vi "main_test.vi"() -> ()   [LabVIEW 2019]
uses:
  <vilib>/myRIO/Instrument Drivers/Onboard IO/I2C/typedefs/I2C Transfer Rate.ctl
  <vilib>/myRIO/Instrument Drivers/Onboard IO/I2C/I2C.lvlib
  <vilib>/myRIO/Instrument Drivers/Onboard IO/I2C/typedefs/I2C User Configuration.ctl
  <vilib>/myRIO/Instrument Drivers/Onboard IO/I2C/typedefs/I2C Configuration.ctl
  <vilib>/myRIO/Common/Instrument Driver Framework/myRIO v1.0/I2C/typedefs/I2C Channels Enum.ctl
  <vilib>/myRIO/Common/Instrument Driver Framework/Utilities/typedefs/Generic FPGA Reference.ctl
  <vilib>/myRIO/Common/Instrument Driver Framework/Utilities/typedefs/myRIO v1.0 Reference.ctl
  <vilib>/myRIO/Common/Instrument Driver Framework/Utilities/typedefs/Hardware Version Enum.ctl
  <vilib>/myRIO/Common/Instrument Driver Framework/Utilities/typedefs/myRIO Generic Hardware Reference.ctl
  <vilib>/myRIO/Instrument Drivers/Onboard IO/I2C/typedefs/I2C Reference.ctl
  <vilib>/myRIO/Instrument Drivers/Onboard IO/I2C/vis/Configure.vi
  <vilib>/userDefined/High Color/nirio_resource_hc.ctl
  <vilib>/myRIO/Common/Instrument Driver Framework/myRIO v1.0/I2C/vis/myRIO v1.1 Open I2C.vi
  <vilib>/myRIO/Instrument Drivers/Onboard IO/I2C/vis/myRIO I2C Open.xnode
  <vilib>/myRIO/Common/Instrument Driver Framework/Utilities/vis/Is FPGA Ref Available.vi
  <vilib>/myRIO/Express VI/Onboard IO/I2C/I2C Express VI.xnode
  <vilib>/Platform/TimedLoop/XDataNode/wakeup.ctl
  <vilib>/Platform/TimedLoop/XDataNode/XDNodeRunTimeDep.lvlib
  <vilib>/Platform/TimedLoop/XDataNode/nitl_modes.ctl
  <vilib>/Platform/TimedLoop/XDataNode/timing_clust.ctl
  <vilib>/platform/TimedLoop/XDataNode/XDataNode.xnode
  <vilib>/myRIO/Instrument Drivers/Onboard IO/I2C/vis/Write.vi
  <vilib>/myRIO/Instrument Drivers/Utilities/Utilities.lvlib
  <vilib>/myRIO/Instrument Drivers/Onboard IO/I2C/vis/Write Read.vi
  <vilib>/myRIO/Express VI/Onboard IO/PWM/PWM Express VI.xnode
  <vilib>/myRIO/Instrument Drivers/Onboard IO/PWM/vis/Set Duty Cycle and Frequency.vi
  <vilib>/myRIO/Instrument Drivers/Onboard IO/PWM/PWM.lvlib
  <vilib>/myRIO/Instrument Drivers/Onboard IO/PWM/typedefs/PWM Configuration.ctl
  <vilib>/myRIO/Common/Instrument Driver Framework/myRIO v1.0/PWM/typedefs/PWM Channels Enum.ctl
  <vilib>/myRIO/Instrument Drivers/Onboard IO/PWM/typedefs/PWM Reference.ctl
  <vilib>/myRIO/Instrument Drivers/Onboard IO/PWM/vis/myRIO PWM Open.xnode
  <vilib>/myRIO/Common/Instrument Driver Framework/myRIO v1.0/PWM/vis/myRIO v1.1 Open PWM.vi
  <vilib>/myRIO/Common/Instrument Driver Framework/myRIO v1.0/DIO/typedefs/DIO Channels Enum.ctl
  <vilib>/myRIO/Common/Instrument Driver Framework/myRIO v1.0/DIO/typedefs/DIO Channels List.ctl
  <vilib>/myRIO/Instrument Drivers/Onboard IO/DIO/typedefs/DIO Reference.ctl
  <vilib>/myRIO/Instrument Drivers/Onboard IO/DIO/DIO.lvlib
  <vilib>/myRIO/Instrument Drivers/Onboard IO/DIO/vis/Write.vi
  <vilib>/myRIO/Common/Instrument Driver Framework/myRIO v1.0/DIO/vis/myRIO v1.1 Open DIO.vi
  <vilib>/myRIO/Instrument Drivers/Onboard IO/DIO/vis/myRIO DIO Open.xnode
  <vilib>/myRIO/Express VI/Onboard IO/DO/DO Express VI.xnode
  <vilib>/imath/engines/lvmath2/RunTimeEngine/BuiltInFunctions/diag/NIMS_diag.vi
  <vilib>/imath/engines/lvmath2/RunTimeEngine/ErrorHandling/NIMS_Create Error From Enums.vi
  <vilib>/imath/engines/lvmath2/RunTimeEngine/NodeEndStatement/NIMS_NodeEndStatement_Output.vi
  <vilib>/imath/engines/lvmath2/RunTimeEngine/ErrorHandling/NIMS_Finalize Error.vi
  <instcachedir>/0/MCStatic_41946317732_460fc674ac509ba7029ac98c4ab25738_40677AF033AE4176B404E9AC0BBDDC84.lvgen/MCStatic_41946317732_460fc674ac509ba7029ac98c4ab25738_40677AF033AE4176B404E9AC0BBDDC84_001.vi
  <instcachedir>/0/MCStatic_41946317732_98df4686c37d1a1eae0c5985e9f7cbe2_A0FFC33B284B421AAD6E5346CB265B3A.lvgen/MCStatic_41946317732_98df4686c37d1a1eae0c5985e9f7cbe2_A0FFC33B284B421AAD6E5346CB265B3A_003.vi
  <instcachedir>/0/MCStatic_41946317732_460fc674ac509ba7029ac98c4ab25738_40677AF033AE4176B404E9AC0BBDDC84.lvgen/MCStatic_41946317732_460fc674ac509ba7029ac98c4ab25738_40677AF033AE4176B404E9AC0BBDDC84_003.vi
  <instcachedir>/0/MCStatic_41946317732_98df4686c37d1a1eae0c5985e9f7cbe2_A0FFC33B284B421AAD6E5346CB265B3A.lvgen/MCStatic_41946317732_98df4686c37d1a1eae0c5985e9f7cbe2_A0FFC33B284B421AAD6E5346CB265B3A_001.vi
  <vilib>/imath/engines/lvmath2/RunTimeEngine/BuiltInFunctions/length/NIMS_length(GV).vi
  <vilib>/imathl/engines/lvmath/Functions/Error Handling/Create Error.vi
  <vilib>/imath/engines/lvmath2/RunTimeEngine/BuiltInFunctions/ones/NIMS_V=ones(I32,I32).vi
  <vilib>/imath/engines/lvmath2/RunTimeEngine/RangeToken/NIMS_Range.vi
  OneDrive/Documents/LabVIEW Data/MathScriptVIs/MCStatic_41946317732_98df4686c37d1a1eae0c5985e9f7cbe2.vi
  <vilib>/imath/engines/lvmath2/RunTimeEngine/ArithmeticOperatorToken/NIMS_ArithmeticOperator_multmx.vi
  <vilib>/imath/engines/lvmath2/RunTimeEngine/BuiltInFunctions/max/1 input/NIMS_max(CM).vi
  <vilib>/imath/engines/lvmath/Functions/Error Handling/MergeErrorsWrapper.vi
  OneDrive/Documents/LabVIEW Data/MathScriptVIs/MCStatic_41946317732_460fc674ac509ba7029ac98c4ab25738.vi
  <vilib>/imath/engines/lvmath2/RunTimeEngine/ArithmeticOperatorToken/NIMS_ArithmeticOperator_minus.vi
  <vilib>/imath/engines/lvmath2/RunTimeEngine/BuiltInFunctions/norm/NIMS_norm(GM,DBL).vi
  <vilib>/imath/engines/lvmath2/RunTimeEngine/BuiltInFunctions/abs/NIMS_abs(signed).vi
  <vilib>/imath/engines/lvmath2/RunTimeEngine/BuiltInFunctions/max/1 input/NIMS_max(RM).vi
  <vilib>/imath/engines/lvmath2/RunTimeSupport/NIMS_Get Scalar_w Error.vi
  <vilib>/imath/engines/lvmath2/RunTimeEngine/BuiltInFunctions/eye/NIMS_M=eye(I32).vi
  <vilib>/imath/engines/lvmath2/RunTimeEngine/ArithmeticOperatorToken/NIMS_ArithmeticOperator_plus.vi
  <vilib>/imath/engines/lvmath2/RunTimeEngine/ArithmeticOperatorToken/NIMS_ArithmeticOperator_leftdivmx(C,C).vi
  <vilib>/imath/engines/lvmath2/RunTimeEngine/ArithmeticOperatorToken/NIMS_ArithmeticOperator_rightdiv.vi
  <vilib>/imath/engines/lvmath2/RunTimeEngine/ArithmeticOperatorToken/NIMS_ArithmeticOperator_rightdivmx(C,C).vi
  <vilib>/imath/engines/lvmath2/RunTimeEngine/ArithmeticOperatorToken/NIMS_ArithmeticOperator_powermx(M,M).vi
  <vilib>/imath/engines/lvmath2/RunTimeEngine/BuiltInFunctions/max/2 inputs/NIMS_max(CG,CG)-no size check.vi
  <vilib>/imath/engines/lvmath2/RunTimeEngine/CommandStatement/MC_CommandStatement_break.vi
  <vilib>/imath/engines/lvmath2/RunTimeEngine/CommandStatement/NIMS_CommandStatement_MaskErr.vi
  <vilib>/imath/engines/lvmath2/RunTimeEngine/NodeEndStatement/NIMS_NodeEndStatement_Get Vector.vi
  <vilib>/imath/engines/lvmath2/RunTimeEngine/BuiltInFunctions/mirrorh/NIMS_mirrorh(GM).vi
  <vilib>/imath/engines/lvmath2/RunTimeEngine/RowToken/NIMS_RowToken_M_M.vi
panel:
  in  "Count(mSec)":u32
  out "XY Graph":cluster{dbl[], dbl[]}[](graph)
  out "pm_hat_opt":dbl[](array[numeric])
  out "Late cycles":u16
  out "B_meas":dbl[](array[numeric])
  in  "Actuation on?":bool
  in  "Slide":dbl(slide) scale=-1.0..1.0
  in  "stop":bool
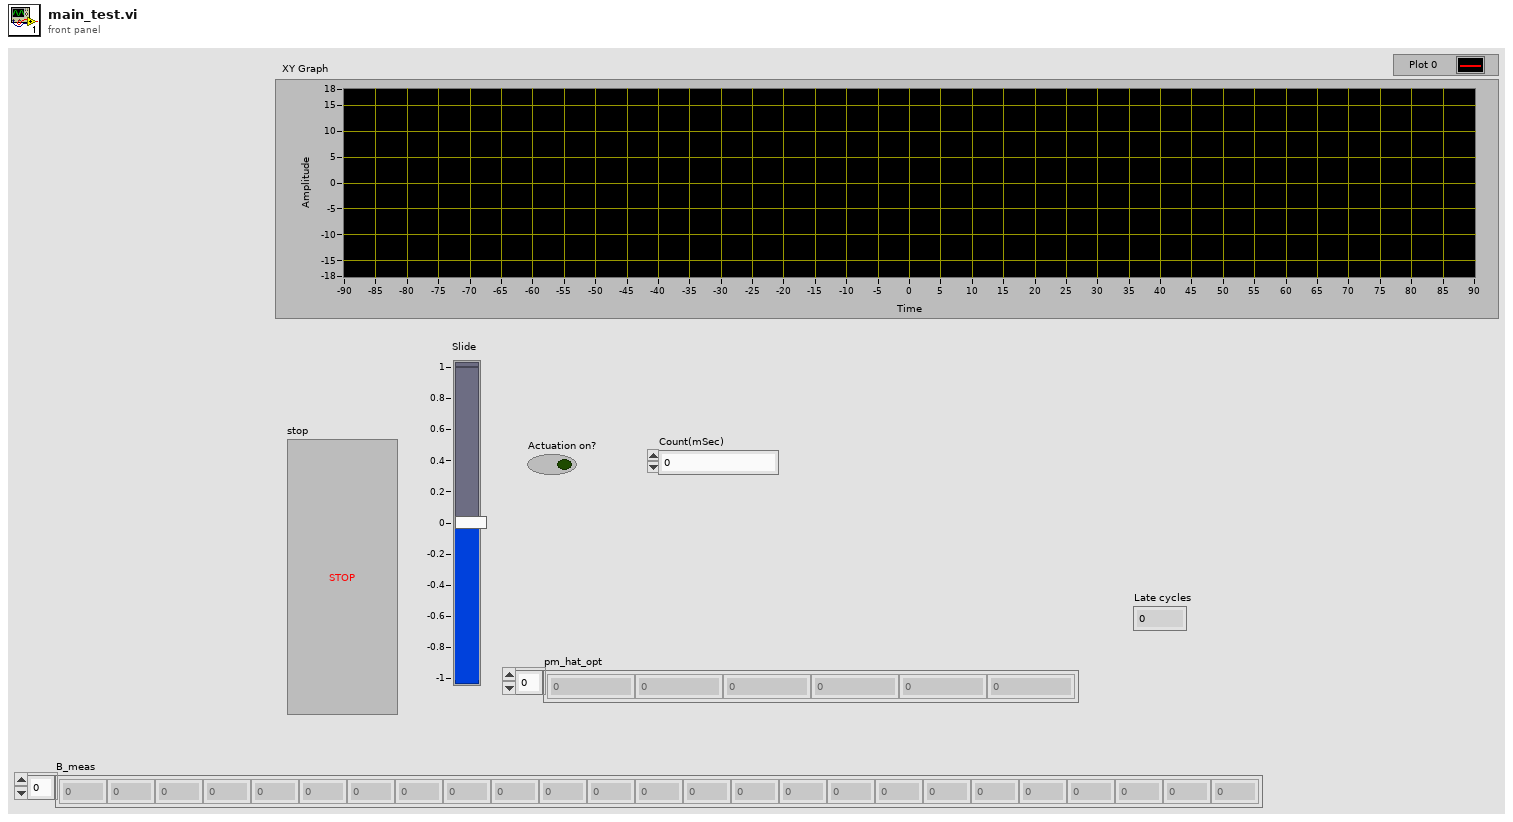
[diagram p1: front panel]
types:
  T1 = typedef "I2C.lvlib/I2C Reference.ctl" = cluster{"myRIO Reference":T2, "I2C Channels Enum":T6, "I2C Configuration":T7}
  T2 = typedef "myRIO Generic Hardware Reference.ctl" = cluster{"myRIO Model":T3, "myRIO Hardware Reference":T4}
  T3 = typedef "Hardware Version Enum.ctl" = enum16{"Unknown", "myRIO-1900", "myRIO-1950", "roboRIO", "NI ELVIS RIO CM", "ELVIS III"}
  T4 = typedef "myRIO v1.0 Reference.ctl" = cluster{"Generic FPGA Reference":T5, "Allow multiple opens":bool}
  T5 = typedef "Generic FPGA Reference.ctl" = refnum<k20>
  T6 = typedef "I2C Channels Enum.ctl" = enum16{"Not Connected", "A/I2C", "B/I2C", "I2C/I2C"}
  T7 = typedef "I2C.lvlib/I2C Configuration.ctl" = cluster{"I2C Transfer Rate":T8}
  T8 = typedef "I2C.lvlib/I2C Transfer Rate.ctl" = enum16{"Standard mode (100 kbps)", "Fast mode (400 kbps)"}
  T9 = typedef "I2C.lvlib/I2C User Configuration.ctl" = cluster{"I2C Transfer Rate":T8}
  T10 = typedef "nirio_resource_hc.ctl" = tag
  T11 = typedef "DIO.lvlib/DIO Reference.ctl" = cluster{"myRIO Reference":T2, "DIO Channels List":T12}
  T12 = typedef "DIO Channels List.ctl" = T13[]
  T13 = typedef "DIO Channels Enum.ctl" = enum16{"Not Connected", "C/DIO0", "C/DIO1", "C/DIO2", "C/DIO3", "C/DIO4", "C/DIO5", "C/DIO6", "C/DIO7", "A/DIO0", "A/DIO1", "A/DIO2", "A/DIO3", "A/DIO4", "A/DIO5", "A/DIO6", "A/DIO7", "A/DIO8", "A/DIO9", "A/DIO10", "A/DIO11", "A/DIO12", "A/DIO13", "A/DIO14", "A/DIO15", "A/DIO16", "A/DIO17", "A/DIO18", "A/DIO19", "B/DIO0", "B/DIO1", "B/DIO2", "B/DIO3", "B/DIO4", "B/DIO5", "B/DIO6", "B/DIO7", "B/DIO8", "B/DIO9", "B/DIO10", "B/DIO11", "B/DIO12", "B/DIO13", "B/DIO14", "B/DIO15", "B/DIO16", "B/DIO17", "B/DIO18", "B/DIO19", "LED0", "LED1", "LED2", "LED3", "Button0", "DIO/DIO0", "DIO/DIO1", "DIO/DIO2", "DIO/DIO3", "DIO/DIO4", "DIO/DIO5", "DIO/DIO6", "DIO/DIO7", "DIO/DIO8", "DIO/DIO9", "SPI/CS0", "SPI/CS1", "SPI/CS2", "SPI/CS3", "LED RADIO (Green)", "LED RADIO (Red)", "LED COMM (Green)", "LED COMM (Red)", "LED MODE (Green)", "LED MODE (Red)"}
  T14 = typedef "PWM.lvlib/PWM Reference.ctl" = cluster{"myRIO Reference":T2, "PWM Channels Enum":T15, "PWM Configuration":T16}
  T15 = typedef "PWM Channels Enum.ctl" = enum16{"Not Connected", "C/PWM0", "C/PWM1", "A/PWM0", "A/PWM1", "A/PWM2", "A/PWM3", "A/PWM4", "A/PWM5", "A/PWM6", "A/PWM7", "A/PWM8", "A/PWM9", "A/PWM10", "A/PWM11", "A/PWM12", "A/PWM13", "A/PWM14", "A/PWM15", "A/PWM16", "A/PWM17", "A/PWM18", "A/PWM19", "B/PWM0", "B/PWM1", "B/PWM2", "B/PWM3", "B/PWM4", "B/PWM5", "B/PWM6", "B/PWM7", "B/PWM8", "B/PWM9", "B/PWM10", "B/PWM11", "B/PWM12", "B/PWM13", "B/PWM14", "B/PWM15", "B/PWM16", "B/PWM17", "B/PWM18", "B/PWM19", "PWM/PWM0", "PWM/PWM1", "PWM/PWM2", "PWM/PWM3", "PWM/PWM4", "PWM/PWM5", "PWM/PWM6", "PWM/PWM7", "PWM/PWM8", "PWM/PWM9"}
  T16 = typedef "PWM.lvlib/PWM Configuration.ctl" = cluster{"Frequency":dbl, "Duty Cycle":dbl}
  T17 = typedef "XDNodeRunTimeDep.lvlib/timing_clust.ctl" = cluster{"Expected End [f-1]":u64, "Actual End [f-1]":u64, "Finished Late? [f-1]":bool, "Expected End [i-1]":u64, "Actual End [i-1]":u64, "Finished Late? [i-1]":bool, "Expected Start [i]":u64, "Actual Start [i]":u64, "Expected Start [f]":u64, "Actual Start [f]":u64, "Source Name":string, "Structure Name":string, "Period":i64, "Deadline":i64, "Offset":i64, "Start":i64, "Priority":i32, "Timeout":i32, "Mode":T18, "Wakeup Reason":T19, "Error":errorcluster, "Source Type":string, "Secondary Source Type":string, "Global End Time":u64, "Global Start Time":u64, "Frame Duration":u64, "Iteration Duration":u64, "Assigned CPU":i32, "I/O Scan Engine Mode":u32}
  T18 = typedef "XDNodeRunTimeDep.lvlib/nitl_modes.ctl" = enum32{"No Change", "Process missed periods, maintain original phase", "Discard missed periods, maintain original phase", "Process missed periods, ignore original phase", "Discard missed periods, ignore original phase"}
  T19 = typedef "XDNodeRunTimeDep.lvlib/wakeup.ctl" = enum32{"Normal", "Aborted", "Asynchronous wakeup", "Timing source error", "Timed loop error", "Timeout"}
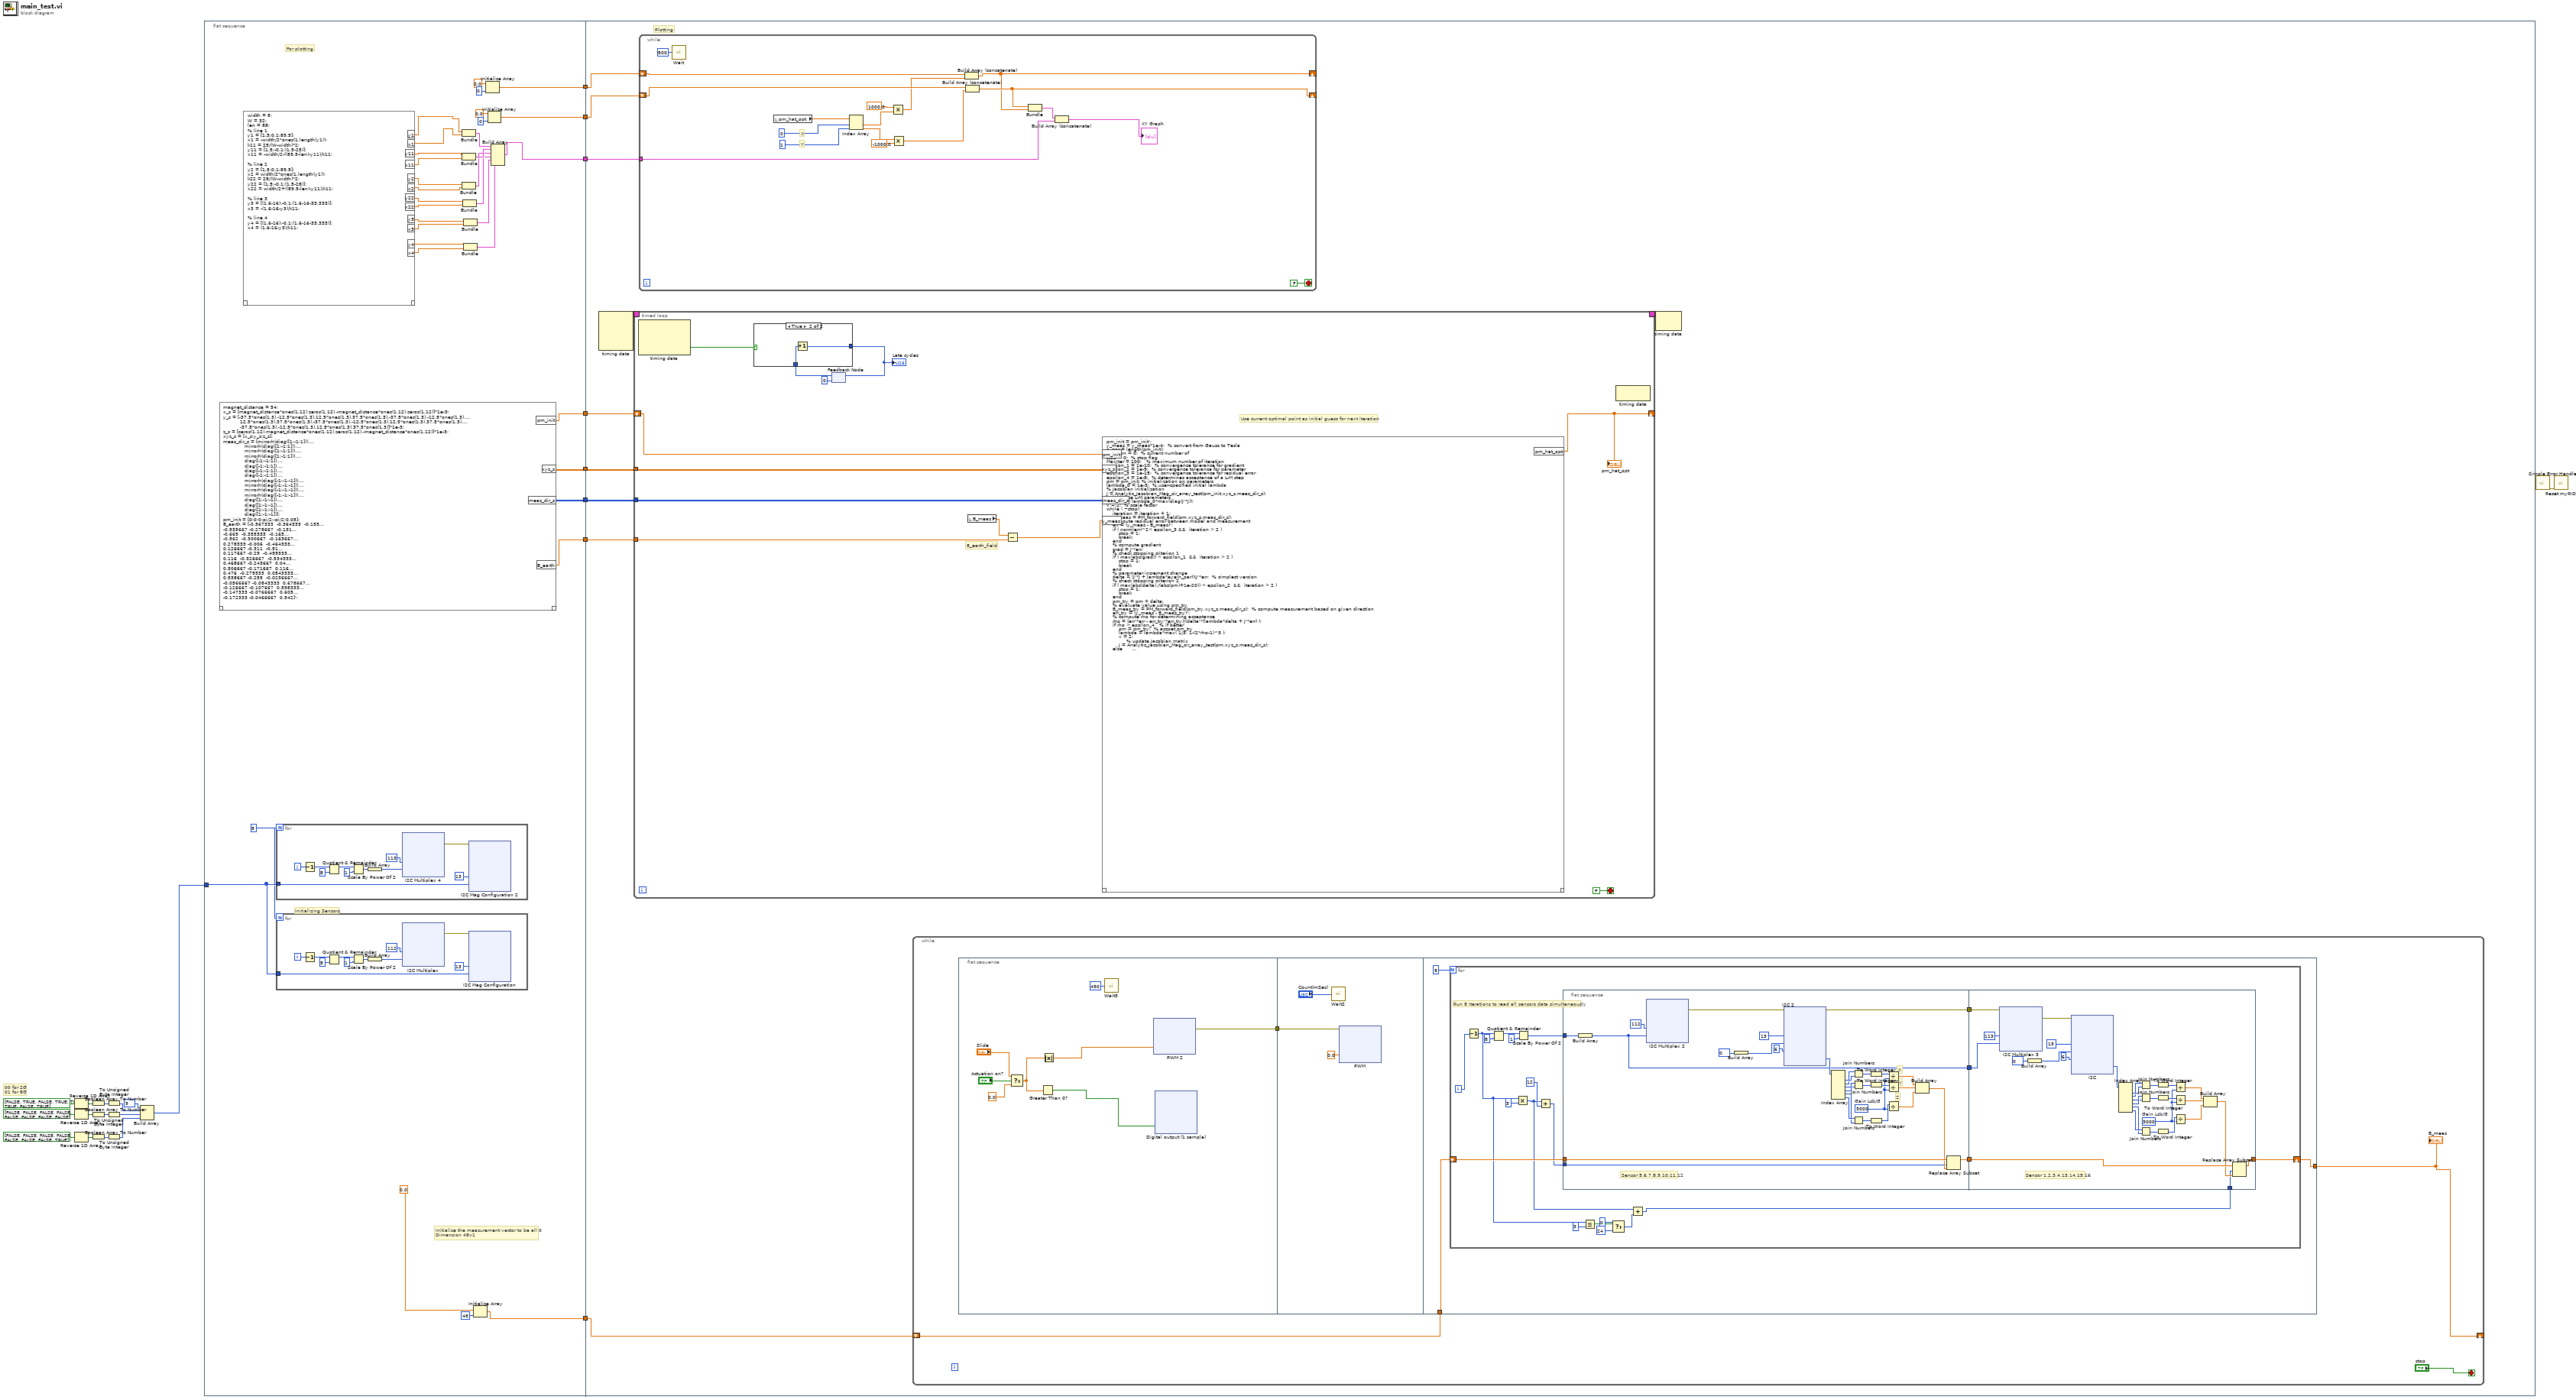
[diagram p0: block diagram]
diagram:
  # "00 for 2G\n01 for 8G"
  n1 = Reverse 1D Array(array=bool[] [FALSE, TRUE, FALSE, TRUE, TRUE, TRUE, FALSE, TRUE]) -> (reversed array=w22:bool[])
  n2 = Reverse 1D Array(array=bool[] [FALSE, FALSE, FALSE, FALSE, FALSE, FALSE, FALSE, FALSE]) -> (reversed array=w21:bool[])
  n3 = Reverse 1D Array(array=bool[] [FALSE, FALSE, FALSE, FALSE, FALSE, FALSE, FALSE, TRUE]) -> (reversed array=w19:bool[])
  n4 = Boolean Array To Number(Boolean array=w22) -> (number=w16:u32)
  n5 = Boolean Array To Number(Boolean array=w21) -> (number=w15:u32)
  n6 = Boolean Array To Number(Boolean array=w19) -> (number=w14:u32)
  n7 = To Unsigned Byte Integer(number=w16) -> (unsigned 8bit integer=w13:u8)
  n8 = To Unsigned Byte Integer(number=w15) -> (unsigned 8bit integer=w12:u8)
  n9 = To Unsigned Byte Integer(number=w14) -> (unsigned 8bit integer=w11:u8)
  n10 = Build Array(u8 9 ("address"), w13, w12, w11) -> (w10:u8[])
  n11 = flat-sequence {
    tunnel: w10 -> [w57]
    tunnel: [w55] -> w8
    tunnel: [w54] -> w7
    tunnel: [w51] -> w6
    tunnel: [w50] -> w5
    tunnel: [w49] -> w4
    tunnel: [w44] -> w3
    tunnel: [w43] -> w2
    tunnel: [w24] -> w1
    tunnel: w8 -> [w784]
    tunnel: w7 -> [w783]
    tunnel: w6 -> [w780]
    tunnel: w5 -> [w779]
    tunnel: w4 -> [w778]
    tunnel: w3 -> [w777]
    tunnel: w2 -> [w776]
    tunnel: w1 -> [w775]
    frame #0 {
      w56 = 8
      # "For plotting"
      # "Initialize the measurement vector to be all 0\nDimension 48x1"
      # "Initializing Sensors"
      n12 = mathscript code="magnet_distance = 54;\nx_s = [magnet_distance*ones(1,12),zeros(1,12),-magnet_distance*ones(1,12),zeros(1,12)]*1e-3; \ny_s = [-37.5*ones(1,3),-12.5*ones(1,3),12.5*ones(1,3),37.5*ones(1,3),-37.5*ones(1,3),-12.5*ones(1,3),...\n           12.5*ones(1,3),37.5*ones(1,3),-37.5*ones(1,3),-12.5*ones(1,3),12.5*ones(1,3),37.5*ones(1,3),...\n           -37.5*ones(1,3),-12.5*ones(1,3),12.5*ones(1,3),37.5*ones(1,3)]*1e-3; \nz_s = [zeros(1,12),magnet_distance*ones(1,12),zeros(1,12),-magnet_distance*ones(1,12)]*1e-3; \nxyz_s = [x_s;y_s;z_s];  \nmeas_dir_s = [mirrorh(diag([1;-1;1])),...\n              mirrorh(diag([1;-1;1])),...\n              mirrorh(diag([1;-1;1])),...\n              mirrorh(diag([1;-1;1])),...\n              diag([-1;-1;1]),...\n              diag([-1;-1;1]),...\n              diag([-1;-1;1]),...\n              diag([-1;-1;1]),...\n              mirrorh(diag([-1;-1;-1])),...\n              mirrorh(diag([-1;-1;-1])),...\n              mirrorh(diag([-1;-1;-1])),...\n              mirrorh(diag([-1;-1;-1])),... \n              diag([1;-1;-1]),...\n              diag([1;-1;-1]),...\n              diag([1;-1;-1]),...\n              diag([1;-1;-1])];\npm_init = [0;0;0;pi/2;-pi/2;0.05];\nB_earth = [-0.567333\t\t-0.364333\t\t-0.155...\n-0.535667\t-0.278667\t\t-0.131...\n-0.669\t\t-0.355333\t\t-0.165...\n-0.562\t\t-0.300667\t\t-0.163667...\n0.278333\t-0.006\t\t-0.464333...\n0.126667\t-0.311\t\t-0.51...\n0.117667\t-0.29\t\t-0.499333...\n0.116\t\t-0.326667\t\t-0.534333...\n0.468667\t-0.243667\t\t0.04...\n0.506667\t-0.171667\t\t0.116...\n0.476\t\t-0.279333\t\t0.0543333...\n0.538667\t-0.255\t\t-0.0236667...\n-0.0566667\t-0.0843333\t\t0.678667...\n-0.126667\t-0.107667\t\t0.598333...\n-0.147333\t-0.0766667\t\t0.605...\n-0.172333\t-0.0466667\t\t0.542]';"() -> ("meas_dir_s"=w55:i32[][], "xyz_s"=w54:dbl[][], "pm_init"=w50:dbl[], "B_earth"=w49:dbl[])  [unwired: 1 in, 1 out]
      n13 = mathscript code="width = 8;\nW = 32;\nlen = 88;\n% line 1\ny1 = [1.5:0.1:89.5];\nx1 = -width/2*ones(1,length(y1));\nk11 = 25/(W-width)*2;\ny11 = [1.5:-0.1:(1.5-25)];\nx11 = -width/2-((89.5-len)-y11)/k11;\n\n% line 2\ny2 = [1.5:0.1:89.5];\nx2 = width/2*ones(1,length(y1));\nk22 = 28/(W-width)*2;\ny22 = [1.5:-0.1:(1.5-28)];\nx22 = width/2+((89.5-len)-y11)/k11;\n\n% line 3\ny3 = [(1.6-16):-0.1:(1.6-16-33.333)];\nx3 = -(1.6-16-y3)/k11;\n\n% line 4\ny4 = [(1.6-16):-0.1:(1.6-16-33.333)];\nx4 = (1.6-16-y3)/k11;"() -> ("y1"=w42:dbl[], "x1"=w41:dbl[], "y11"=w40:dbl[], "x11"=w39:dbl[], "y2"=w36:dbl[], "x2"=w35:dbl[], "y22"=w33:dbl[], "x22"=w32:dbl[], "y3"=w30:dbl[], "x3"=w29:dbl[], "y4"=w27:dbl[], "x4"=w26:dbl[])  [unwired: 1 in, 1 out]
      n14 = for {
        N: w56 -> [_]
        tunnel: w57 -> [w608]
        i -> [w602]
        n15 = Decrement(x=w602) -> (x-1=w601:i32)
        n16 = Quotient & Remainder(x=w601, y=8) -> (x-y*floor(x/y)=w603:i32)  [unwired: 1 out]
        n17 = Scale By Power Of 2(n=w603, x=1) -> (x*2^n=w605:i32)
        n18 = Build Array(w605) -> (w611:i32[])
        n19 = xnode "I2C Multiplex 4"("Slave Address (7-bit)"=u8 113, "Bytes to Write"=w611) -> ("error out"=w610:errorcluster)  [unwired: 1 in]
        n20 = xnode "I2C Mag Configuration 2"("Slave Address (7-bit)"=u8 13, "Bytes to Write"=w608, "error in (no error)"=w610) -> ()  [unwired: 1 out]
      }
      n21 = for {
        N: w56 -> [_]
        tunnel: w57 -> [w695]
        i -> [w689]
        n22 = Decrement(x=w689) -> (x-1=w688:i32)
        n23 = Quotient & Remainder(x=w688, y=8) -> (x-y*floor(x/y)=w690:i32)  [unwired: 1 out]
        n24 = Scale By Power Of 2(n=w690, x=1) -> (x*2^n=w692:i32)
        n25 = Build Array(w692) -> (w698:i32[])
        n26 = xnode "I2C Multiplex"("Slave Address (7-bit)"=u8 112, "Bytes to Write"=w698) -> ("error out"=w697:errorcluster)  [unwired: 1 in]
        n27 = xnode "I2C Mag Configuration"("Slave Address (7-bit)"=u8 13, "Bytes to Write"=w695, "error in (no error)"=w697) -> ()  [unwired: 1 out]
      }
      n28 = Bundle("y2"=w36, "x2"=w35) -> (w34:cluster{"y2":dbl[], "x2":dbl[]})  [unwired: 1 in]
      n29 = Bundle("y1"=w42, "x1"=w41) -> (w38:cluster{"y1":dbl[], "x1":dbl[]})  [unwired: 1 in]
      n30 = Bundle("y11"=w40, "x11"=w39) -> (w37:cluster{"y11":dbl[], "x11":dbl[]})  [unwired: 1 in]
      n31 = Bundle("y22"=w33, "x22"=w32) -> (w31:cluster{"y22":dbl[], "x22":dbl[]})  [unwired: 1 in]
      n32 = Bundle("y3"=w30, "x3"=w29) -> (w28:cluster{"y3":dbl[], "x3":dbl[]})  [unwired: 1 in]
      n33 = Bundle("y4"=w27, "x4"=w26) -> (w25:cluster{"y4":dbl[], "x4":dbl[]})  [unwired: 1 in]
      n34 = Initialize Array(0.0 ("element"), 48 ("dimension size")) -> (w51:dbl[])
      n35 = Initialize Array(0.0 ("element"), 0 ("dimension size")) -> (w44:dbl[])
      n36 = Initialize Array(0.0 ("element"), 0 ("dimension size")) -> (w43:dbl[])
      n37 = Build Array(w38, w37, w34, w31, w28, w25) -> (w24:cluster{"y4":dbl[], "x4":dbl[]}[])
    }
    frame #1 {
      # "Plotting"
      n38 = node-c288() -> (w782:T17)  [unwired: 4 in]
      n39 = timed-loop {
        tunnel: w784 -> [w1173]
        tunnel: w783 -> [w1172]
        timing: w782 -> [_]
        timing-out: [_] -> w781
        shift-right: [w1165] -> _
        shift-left: w779 -> [w1166]
        tunnel: w778 -> [w1163]
        stop <- FALSE stop-if-true
        # "B_earth_field"
        # "Use current optimal point as initial guess for next iteration"
        n40 = node-c288() -> (w1167:bool)  [unwired: 1 in, 3 out]
        n41 = feedback #1(u16 0) -> (w1170:u16)
        n42 = case shown="True" w1167 {
          tunnel: w1170 -> [w1174 w1176]
          tunnel: [w1174 w1175] -> w1169
          frame False {
          }
          frame True {
            n43 = Increment(x=w1176) -> (x+1=w1175:u16)
          }
        }
        "Late cycles" <- w1169
        n44 = feedback-in #1(w1169) -> ()
        n45 = local read "B_meas"() -> (w1164:dbl[])
        n46 = Subtract(x=w1164, y=w1163) -> (x-y=w1162:dbl[])
        n47 = mathscript code="pm_init = pm_init';\ny_meas = y_meas*1e-4;  % convert from Gauss to Tesla\nn_par = length(pm_init);\niteration = 0;  % current number of \nstop = 0;  % stop flag\nMaxIter = 100;   % maximum number of iteration\nepsilon_1 = 1e-10;  % convergence tolerance for gradient\nepsilon_2 = 1e-9;  % convergence tolerance for parameter\nepsilon_3 = 1e-15;  % convergence tolerance for residual error\nepsilon_4 = 1e-8;  % determines acceptance of a L-M step\npm = pm_init; % initialization on parameters\nlambda_0 = 1e-3;  % user-specified initial lambda\n% Jacobian initialization\nJ = Analytic_Jacobian_Mag_cir_array_test(pm_init,xyz_s,meas_dir_s);\n% initialize L-M parameters\nlambda = lambda_0*max(diag(J'*J));\nv = 2;  % scale factor\nwhile ( ~stop)\n    iteration = iteration + 1;\n    B_meas = PM_forward_field(pm,xyz_s,meas_dir_s);\n% compute residual error between model and measurement\n    err = (y_meas - B_meas)';\n    if ( norm(err)^2< epsilon_3 &&  iteration > 2 )\n        stop = 1;\n        break;\n    end\n    % compute gradient\n    grad = J'*err;\n    % check stopping criterion 1\n    if ( max(abs(grad)) < epsilon_1  &&  iteration > 2 )\n        stop = 1;\n        break\n    end\n    % parameter increment change\n    delta = (J'*J + lambda*eye(n_par))\\J'*err;  % simplest version\n    % check stopping criterion 2 \n    if ( max(abs(delta)./(abs(pm)+1e-20)) < epsilon_2  &&  iteration > 2 )\n        stop = 1;\n        break\n    end\n    pm_try = pm + delta;\n    % evaluate value using pm_try\n    B_meas_try = PM_forward_field(pm_try,xyz_s,meas_dir_s);  % compute measurement based on given direction\n    err_try = (y_meas - B_meas_try)';\n    % compute rho for determining acceptance\n    rho = (err'*err - err_try'*err_try)/(delta'*(lambda*delta + J'*err) );\n    if rho > epsilon_4   % if better\n        pm = pm_try;  % accpet pm_try\n        lambda = lambda*max( 1/3, 1-(2*rho-1)^3 );\n        v = 2;\n             % update Jacobian matrix\n        J = Analytic_Jacobian_Mag_cir_array_test(pm,xyz_s,meas_dir_s);\n    else      % if not better\n        lambda = lambda*v;\n        v = 2*v;\n    end\n    if ( iteration == MaxIter )\n        stop = 1;\n    end\nend\n\npm_hat_opt = pm;"("meas_dir_s"=w1173, "xyz_s"=w1172, "y_meas"=w1162, "pm_init"=w1166) -> ("pm_hat_opt"=w1165:dbl[])  [unwired: 1 in, 1 out]
        "pm_hat_opt" <- w1165
        n48 = node-c288() -> ()  [unwired: 1 in, 1 out]
      }
      n49 = while {
        shift-right: [w1153] -> _
        shift-left: w777 -> [w1156]
        shift-right: [w1154] -> _
        shift-left: w776 -> [w1155]
        tunnel: w775 -> [w1144]
        stop <- FALSE stop-if-true
        # "X"
        # "Y"
        n50 = call "Wait"("Count(mSec)"=u32 500) -> ()  [unwired: 1 out]
        n51 = local read "pm_hat_opt"() -> (w1160:dbl[])
        n52 = Index Array(array=w1160, index #1=0 ("index"), index #2=1 ("index")) -> (element #1=w1149:dbl, element #2=w1152:dbl)
        n53 = Multiply(x=1000.0, y=w1149) -> (x*y=w1147:dbl)
        n54 = Multiply(x=w1152, y=-1000.0) -> (x*y=w1150:dbl)
        n55 = Build Array (concatenate)(w1156, w1147) -> (w1153:dbl[])
        n56 = Build Array (concatenate)(w1155, w1150) -> (w1154:dbl[])
        n57 = Bundle(w1154, w1153) -> (w1145:cluster{dbl[], dbl[]})  [unwired: 1 in]
        n58 = Build Array (concatenate)(w1145, w1144) -> (→"XY Graph":cluster{"y4":dbl[], "x4":dbl[]}[])
      }
      n59 = while {
        shift-right: [w785] -> _
        shift-left: w780 -> [w786]
        stop <- "stop" stop-if-true
        n60 = flat-sequence {
          tunnel: [w795] -> w787
          tunnel: w787 -> [w868]
          tunnel: w786 -> [w906]
          tunnel: [w905] -> w785
          frame #0 {
            n61 = Select(t="Slide", s="Actuation on?", f=0.0) -> (s? t:f=w790:dbl)
            n62 = Greater Than 0?(x=w790) -> (x > 0?=w789:bool)
            n63 = Absolute Value(x=w790) -> (abs(x)=w791:dbl)
            n64 = call "Wait3"("Count(mSec)"=u32 490) -> ()  [unwired: 1 out]
            n65 = xnode "PWM 2"("Duty Cycle"=w791) -> ("error out"=w795:errorcluster)  [unwired: 1 in]
            n66 = xnode "Digital output (1 sample)"("C/DIO2 (DIO2)"=w789) -> ()  [unwired: 1 in, 1 out]
          }
          frame #1 {
            n67 = call "Wait2"("Count(mSec)"="Count(mSec)") -> ()  [unwired: 1 out]
            n68 = xnode "PWM"("Duty Cycle"=0.0, "error in (no error)"=w868) -> ()  [unwired: 1 out]
          }
          frame #2 {
            # "Run 8 Iterations to read all sensors data simultaneously"
            n69 = for {
              N: 8 -> [_]
              shift-right: [w919] -> w905
              shift-left: w906 -> [w921]
              i -> [w922]
              n70 = Decrement(x=w922) -> (x-1=w915:i32)
              n71 = Quotient & Remainder(x=w915, y=8) -> (x-y*floor(x/y)=w923:i32)  [unwired: 1 out]
              n72 = Multiply(x=w915, y=3) -> (x*y=w912:i32)
              n73 = Scale By Power Of 2(n=w923, x=1) -> (x*2^n=w924:i32)
              n74 = Add(x=w912, y=12) -> (x+y=w916:i32)
              n75 = flat-sequence {
                tunnel: w926 -> [w939]
                tunnel: [w939] -> w929
                tunnel: [w937] -> w928
                tunnel: w921 -> [w933]
                tunnel: [w932] -> w920
                tunnel: w916 -> [w930]
                tunnel: w929 -> [w1046]
                tunnel: w928 -> [w1044]
                tunnel: w920 -> [w1043]
                tunnel: [w1042] -> w919
                tunnel: w908 -> [w1037]
                frame #0 {
                  w948 = i16 3000  # Gain Lsb/G
                  # "Sensor 5,6,7,8,9,10,11,12"
                  # "Z"
                  # "Y"
                  # "X"
                  n76 = xnode "I2C Multiplex 2"("Slave Address (7-bit)"=u8 112, "Bytes to Write"=w939) -> ("error out"=w938:errorcluster)  [unwired: 1 in]
                  n77 = Build Array(u8 0) -> (w952:u8[])
                  n78 = xnode "I2C 2"("Slave Address (7-bit)"=u8 13, "Bytes to Write"=w952, "Byte Count"=u32 6, "error in (no error)"=w938) -> ("Bytes Read"=w955:u8[], "error out"=w937:errorcluster)
                  n79 = Index Array(array=w955) -> (element #1=w947:u8, element #2=w946:u8, element #3=w944:u8, element #4=w945:u8, element #5=w942:u8, element #6=w943:u8)  [unwired: 6 in]
                  n80 = Join Numbers(hi=w946, lo=w947) -> ((hi.lo)=w958:u16)
                  n81 = Join Numbers(hi=w945, lo=w944) -> ((hi.lo)=w956:u16)
                  n82 = Join Numbers(hi=w943, lo=w942) -> ((hi.lo)=w957:u16)
                  n83 = To Word Integer(number=w958) -> (16bit integer=w951:i16)
                  n84 = To Word Integer(number=w956) -> (16bit integer=w950:i16)
                  n85 = To Word Integer(number=w957) -> (16bit integer=w949:i16)
                  n86 = Divide(x=w951, y=w948) -> (x/y=w936:dbl)
                  n87 = Divide(x=w950, y=w948) -> (x/y=w935:dbl)
                  n88 = Divide(x=w949, y=w948) -> (x/y=w934:dbl)
                  n89 = Build Array(w936, w935, w934) -> (w931:dbl[])
                  n90 = Replace Array Subset(array=w933, new element=w931, index=w930) -> (w932:dbl[])
                }
                frame #1 {
                  w1055 = i16 3000  # Gain Lsb/G
                  # "Sensor 1,2,3,4,13,14,15,16"
                  n91 = xnode "I2C Multiplex 3"("Slave Address (7-bit)"=u8 113, "Bytes to Write"=w1046, "error in (no error)"=w1044) -> ("error out"=w1045:errorcluster)
                  n92 = Build Array(u8 0) -> (w1059:u8[])
                  n93 = xnode "I2C"("Slave Address (7-bit)"=u8 13, "Bytes to Write"=w1059, "Byte Count"=u32 6, "error in (no error)"=w1045) -> ("Bytes Read"=w1062:u8[])  [unwired: 1 out]
                  n94 = Index Array(array=w1062) -> (element #1=w1054:u8, element #2=w1053:u8, element #3=w1051:u8, element #4=w1052:u8, element #5=w1049:u8, element #6=w1050:u8)  [unwired: 6 in]
                  n95 = Join Numbers(hi=w1053, lo=w1054) -> ((hi.lo)=w1065:u16)
                  n96 = Join Numbers(hi=w1052, lo=w1051) -> ((hi.lo)=w1063:u16)
                  n97 = Join Numbers(hi=w1050, lo=w1049) -> ((hi.lo)=w1064:u16)
                  n98 = To Word Integer(number=w1065) -> (16bit integer=w1058:i16)
                  n99 = To Word Integer(number=w1063) -> (16bit integer=w1057:i16)
                  n100 = To Word Integer(number=w1064) -> (16bit integer=w1056:i16)
                  n101 = Divide(x=w1058, y=w1055) -> (x/y=w1041:dbl)
                  n102 = Divide(x=w1057, y=w1055) -> (x/y=w1040:dbl)
                  n103 = Divide(x=w1056, y=w1055) -> (x/y=w1039:dbl)
                  n104 = Build Array(w1041, w1040, w1039) -> (w1038:dbl[])
                  n105 = Replace Array Subset(array=w1043, new element=w1038, index=w1037) -> (w1042:dbl[])
                }
              }
              n106 = Build Array(w924) -> (w926:i32[])
              n107 = Less Or Equal?(x=w915, y=3) -> (x <= y?=w913:bool)
              n108 = Select(t=0, s=w913, f=24) -> (s? t:f=w909:i32)
              n109 = Add(x=w912, y=w909) -> (x+y=w908:i32)
            }
          }
        }
        "B_meas" <- w785
      }
      n110 = node-c288(w781) -> ()  [unwired: 1 out]
    }
  }
  n111 = call <vilib>:"Simple Error Handler.vi"() -> ("error out"=w9:errorcluster)  [unwired: 5 in, 4 out]
  n112 = call <vilib>:"Reset myRIO.vi"("error in (no error)"=w9) -> ()  [unwired: 10 in, 1 out]
